vi "Handle Error.vi"(8 "error in (no error)":errorcluster, 11 "UI_Actor in":refnum<class "UI_Actor.lvclass">) -> (0 "error out":errorcluster, 2 "stop actor?":bool=TRUE, 3 "UI_Actor out":refnum<class "UI_Actor.lvclass">)   [LabVIEW 2020, in "UI_Actor.lvlib" / "UI_Actor.lvclass"]
doc: "(<B>Filename</B>: Actor Framework.lvlib:Actor.lvclass:Handle Error.vi)\n\nDefines how the actor handles an error that occurred while processing a message. By default, this method does nothing except stop the actor."
uses:
  UI_Actor.lvclass
  D:/Projets/STEP AT/UI Actor/support/Actor Framework.lvlibp/1abvi3w/vi.lib/ActorFramework/Actor/Actor.lvclass
  UI_Actor.lvclass/UI_Actor.ctl
  support/Actor Framework.lvlibp/1abvi3w/vi.lib/ActorFramework/Actor/Actor.lvclass
  support/Actor Framework.lvlibp/1abvi3w/vi.lib/ActorFramework/Report Error Msg/Report Error Msg.lvclass
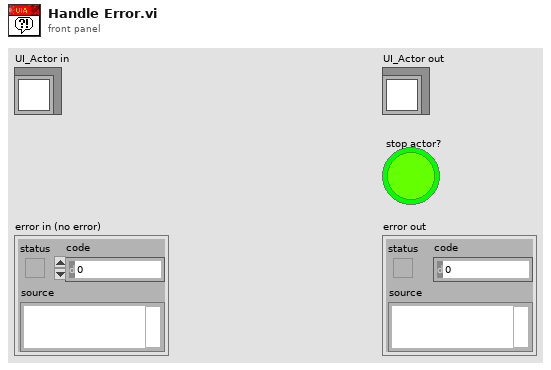
[diagram p1: front panel]
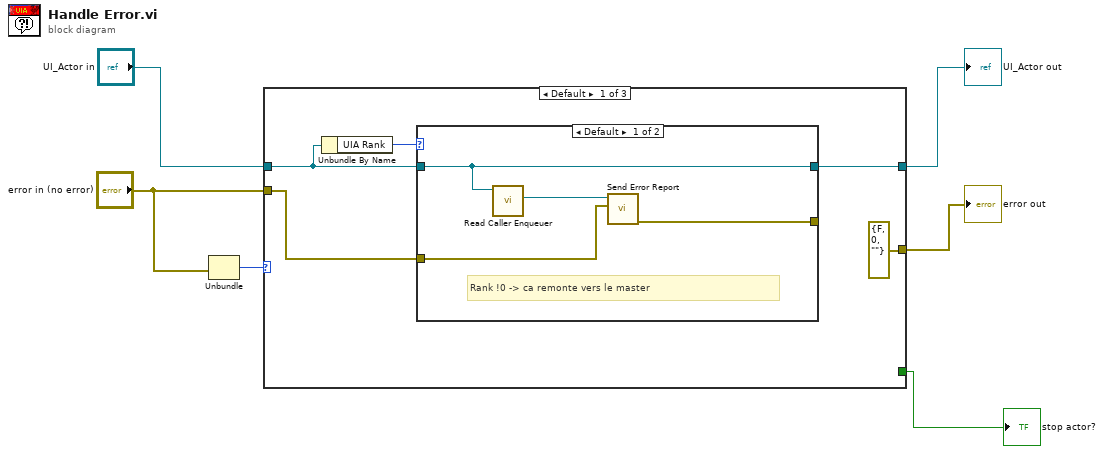
[diagram p0: block diagram]
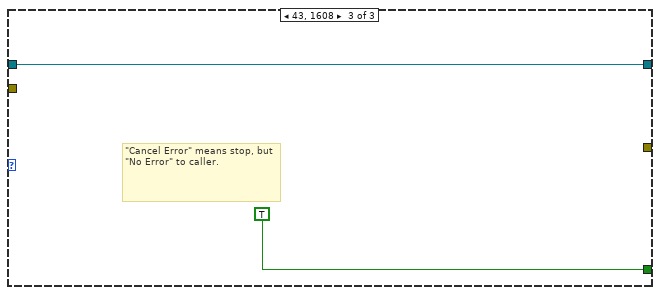
[diagram p4: hidden frame]
diagram:
  n1 = Unbundle("error in (no error)") -> ("code"=w6:i32)  [unwired: 2 out]
  n2 = case shown="Default" w6 {
    tunnel: [errorcluster {"status"=FALSE, "code"=0, "source"=""} ("error in (no error)") _ _] -> w3
    tunnel: "error in (no error)" -> [w7 _ _]
    tunnel: [_ _ TRUE] -> w5
    tunnel: "UI_Actor in" -> [w9 w18 w19]
    tunnel: [w8 w18 w19] -> w1
    frame Default {
      n3 = Unbundle By Name(w9) -> ("UIA Rank"=w10:i32)
      n4 = case shown="Default" w10 {
        tunnel: [w15 w17] -> w8
        tunnel: w9 -> [w15 w17]
        tunnel: [w12 w16] -> _
        tunnel: w7 -> [w13 w16]
        frame Default {
          # "Rank !0 -> ca remonte vers le master"
          n5 = call "Read Caller Enqueuer.vi"("Actor"=w15) -> ("Caller Enqueuer"=w14:refnum<class "Message Enqueuer.lvclass">)  [unwired: 10 in]
          n6 = call "Send Error Report.vi"("Error From Sender"=w13, "Message Enqueuer"=w14) -> ("error out"=w12:errorcluster)  [unwired: 9 in]
        }
        frame 0 {
          # "Rank 0 -> On est le master.\n=> Il faut faire un override de ce VI\net gérer l'erreur ici"
        }
      }
    }
    frame 0 {
    }
    frame 43, 1608 {
      # "\"Cancel Error\" means stop, but \"No Error\" to caller."
    }
  }
  "UI_Actor out" <- w1
  "error out" <- w3
  "stop actor?" <- w5
